vi "暫存.vi"() -> ()   [LabVIEW 2020]
panel:
  out "Reference Path":waveform(dbl)(graph)
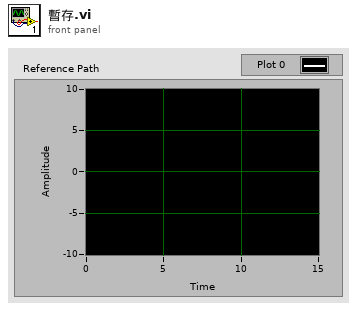
[diagram p1: front panel]
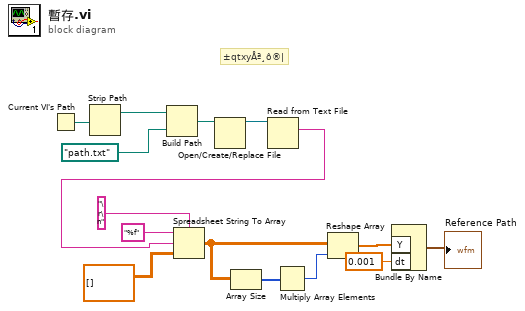
[diagram p0: block diagram]
diagram:
  # "±qtxyÅª¸ô®|"
  n1 = Current VI's Path() -> (path=w15:path)
  n2 = Strip Path(path=w15) -> (stripped path=w14:path)  [unwired: 1 out]
  n3 = Build Path(base path=w14, name or relative path=path "path.txt") -> (appended path=w12:path)
  n4 = Open/Create/Replace File(file path (use dialog)=w12) -> (refnum out=w11:refnum<file>)  [unwired: 5 in, 2 out]
  n5 = Read from Text File(file (use dialog)=w11) -> (text=w8:string)  [unwired: 3 in, 3 out]
  n6 = Spreadsheet String To Array(delimiter (Tab)="\r\n", format string="%f", spreadsheet string=w8, array type (2D Dbl)=dbl[][] []) -> (array=w6:dbl[][])
  n7 = Array Size(array=w6) -> (size(s)=w5:i32[])
  n8 = Multiply Array Elements(1:w5) -> (0:w4:i32)
  n9 = Reshape Array(w6, w4) -> (w1:dbl[])
  n10 = Bundle By Name("Y"=w1, "dt"=0.001) -> (→"Reference Path":waveform(dbl))  [unwired: 1 in]
